vi "ReplyToViewer.vi"(8 "error in (no error)":errorcluster, 10 "ReplyToViewer":T1, 11 "Gserver in":refnum<class "Gserver.lvclass">) -> (0 "error out":errorcluster, 3 "Gserver out":refnum<class "Gserver.lvclass">)   [LabVIEW 2020, in "Sgraph_lib_V1.lvlib" / "Gserver.lvclass"]
doc: "Andre Koelewijn, 1-7-2023\n\nSend data back to one graph viewer"
uses:
  Gserver.lvclass
  controls/Typedef_ReplyToViewer.ctl
  Gview/controls/Typedef_Gserver-Replies.ctl
  Gview/controls/Typedef_ServerActions.ctl
  Gserver.lvclass/Gserver.ctl
  Builds/Sgraph_lib_V1.lvlib
  Gview/Gviewer.lvclass
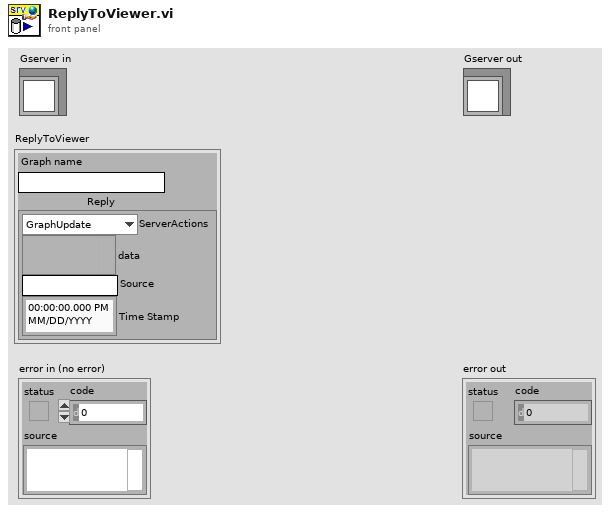
[diagram p1: front panel]
types:
  T1 = typedef "Typedef_ReplyToViewer.ctl" = cluster{"Graph name":string, "Reply":T2}
  T2 = typedef "Typedef_Gserver-Replies.ctl" = cluster{"ServerActions":T3, "data":variant, "Source":string, "Time Stamp":timestamp}
  T3 = typedef "Sgraph_lib_V1.lvlib/Gviewer.lvclass/Typedef_ServerActions.ctl" = enum16{"GraphUpdate", "SendAllTags", "SendIniPath", "SetGeneralOptions", "EditTagsOpen", "EditTagsPresetSave", "EditTagsPresetLoad", "EditTagsClose", "NewTagSelection", "AutoScale", "DBeditStatus", "DBsaveConfirm", "GetXconstraints", "ExitGraph"}
  T4 = typedef "Sgraph_lib_V1.lvlib/Gserver.lvclass/Typedef_Sgraph_Query.ctl" = cluster{"ViewportName":string, "Tags":string[], "Time-Start":timestamp, "Time-End":timestamp, "Pixels":i32, "Live":T5, "TimeSpan(sec)":dbl, "GViewer-Queue":refnum<queue>, "Network":bool, "IP-address":string, "Port":u16, "connection-ID":refnum<k5>, "TCP-buffer":string}
  T5 = typedef "Sgraph_lib_V1.lvlib/Gviewer.lvclass/Typedef_Live.ctl" = enum16{"Live View", "Freeze"}
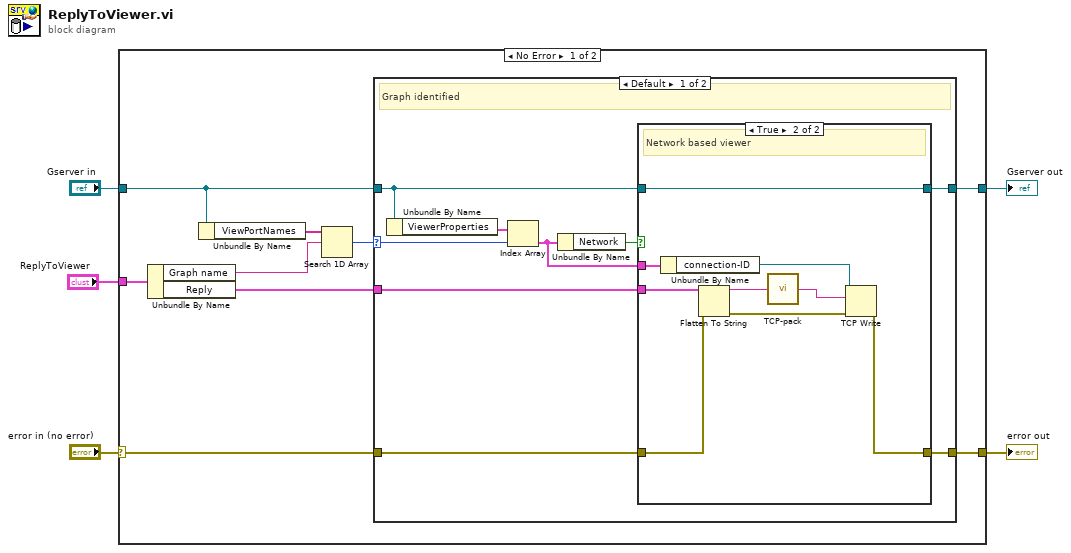
[diagram p0: block diagram]
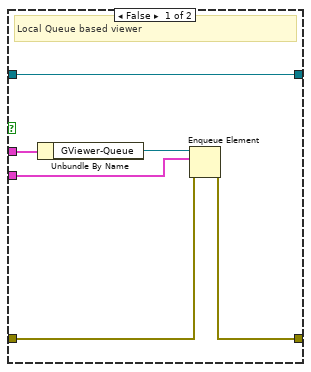
[diagram p2: hidden frame]
diagram:
  n1 = case shown="No Error" "error in (no error)" {
    selector: "error in (no error)" -> [w10 w42]
    tunnel: [w9 w42] -> w4
    tunnel: [w11 w41] -> w2
    tunnel: "Gserver in" -> [w12 w41]
    tunnel: "ReplyToViewer" -> [w8 _]
    frame No Error {
      n2 = Unbundle By Name(w8) -> ("Graph name"=w7:string, "Reply"=w6:T2)
      n3 = Unbundle By Name(w12) -> ("ViewPortNames"=w14:string[])
      n4 = Search 1D Array(1D array=w14, element=w7) -> (index of element=w13:i32)  [unwired: 1 in]
      n5 = case shown="Default" w13 {
        selector: w13 -> [w22 _]
        tunnel: w12 -> [w20 w40]
        tunnel: [w17 w40] -> w11
        tunnel: w10 -> [w19 w39]
        tunnel: [w18 w39] -> w9
        tunnel: w6 -> [w16 _]
        frame Default {
          # "Graph identified"
          n6 = Unbundle By Name(w20) -> ("ViewerProperties"=w23:T4[])
          n7 = Index Array(array=w23, index=w22) -> (element=w15:T4)
          n8 = Unbundle By Name(w15) -> ("Network"=w21:bool)
          n9 = case shown="True" w21 {
            tunnel: w20 -> [w26 w37]
            tunnel: w19 -> [w28 w31]
            tunnel: [w27 w30] -> w18
            tunnel: [w26 w37] -> w17
            tunnel: w16 -> [w25 w36]
            tunnel: w15 -> [w24 w38]
            frame False {
              # "Local Queue based viewer"
              n10 = Unbundle By Name(w24) -> ("GViewer-Queue"=w29:refnum<queue>)
              n11 = Enqueue Element(queue=w29, element=w25, error in (no error)=w28) -> (error out=w27:errorcluster)  [unwired: 1 in, 2 out]
            }
            frame True {
              # "Network based viewer"
              n12 = Unbundle By Name(w38) -> ("connection-ID"=w34:refnum<k5>)
              n13 = Flatten To String(anything=w36, error in (no error)=w31) -> (data string=w35:string, error out=w33:errorcluster)  [unwired: 2 in, 1 out]
              n14 = call "TCP-pack.vi"("Data to send"=w35) -> ("Data toTCP"=w32:string)  [unwired: 6 in]
              n15 = TCP Write(connection ID=w34, data in=w32, error in (no error)=w33) -> (error out=w30:errorcluster)  [unwired: 1 in, 2 out]
            }
          }
        }
        frame -1 {
          # "graph name not found"
        }
      }
    }
    frame Error {
    }
  }
  "error out" <- w4
  "Gserver out" <- w2
